vi "cam5_3dTest.vi"(7 "park plane z (px)":dbl=100.0, 8 "3d graph":refnum<k7>, 9 "transform cluster + actuator":T1, 10 "positions":T2, 11 "cells (image px locations)":dbl[][](array[numeric])=[[100.0, 300.0], [200.0, 400.0]]) -> (0 "current stage location (px)":dbl[](array[numeric]), 1 "current pipette locations (px)":dbl[][](array[numeric]), 2 "current cell locations (px)":dbl[][](array[numeric]), 3 "currentState out":T3(array[cluster]), 5 "current park plane z (px)":dbl=100.0)   [LabVIEW 2015]
uses:
  pipette cleaning/pressure box/cleaning_soft/controls/actuator_type.ctl
  pipette cleaning/pressure box/cleaning_soft/controls/actuator_cluster.ctl
  controls/transform_cluster_actuator.ctl
  transform_properties_actuators.ctl
panel:
  # "9/12/16\nUPDATES\n- real flag: show manipulator only if they are real"
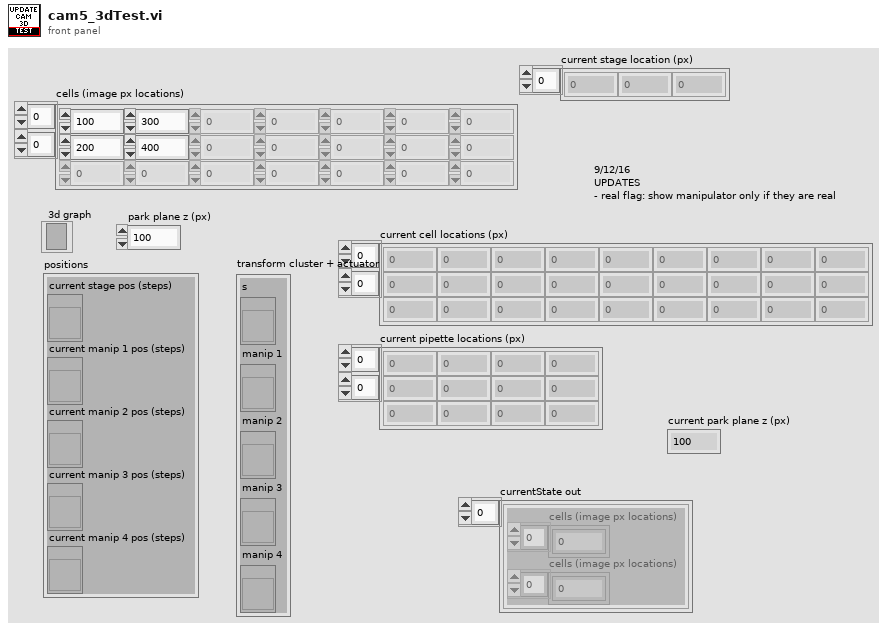
[diagram p1: front panel]
types:
  T1 = typedef "transform_cluster_actuator.ctl" = cluster{"s":refnum<vi>, "manip 1":refnum<vi>, "manip 2":refnum<vi>, "manip 3":refnum<vi>, "manip 4":refnum<vi>}
  T2 = cluster{"current stage pos (steps)":refnum<vi>, "current manip 1 pos (steps)":refnum<vi>, "current manip 2 pos (steps)":refnum<vi>, "current manip 3 pos (steps)":refnum<vi>, "current manip 4 pos (steps)":refnum<vi>}
  T3 = cluster{"cells (image px locations)":dbl[], "cells (image px locations)":dbl[]}[]
  T4 = typedef "transform_properties_actuators.ctl" = cluster{"theta (deg)":dbl, "X sc factor (px/step)":dbl, "Y sc factor (px/step)":dbl, "zero loc (x,y,z)":dbl[], "flip y?":bool, "flip x?":bool, "gamma (deg)":dbl, "flip z?":bool, "Z sc factor (px/step)":dbl, "actuator":T5, "safe space (steps)":i32[]}
  T5 = typedef "actuator_cluster.ctl" = cluster{"Actuator COM":refnum<visa-resource-name>, "Actuator type":T6}
  T6 = typedef "actuator_type.ctl" = enum16{"Scientifica", "Sutter", "Demo", "Off"}
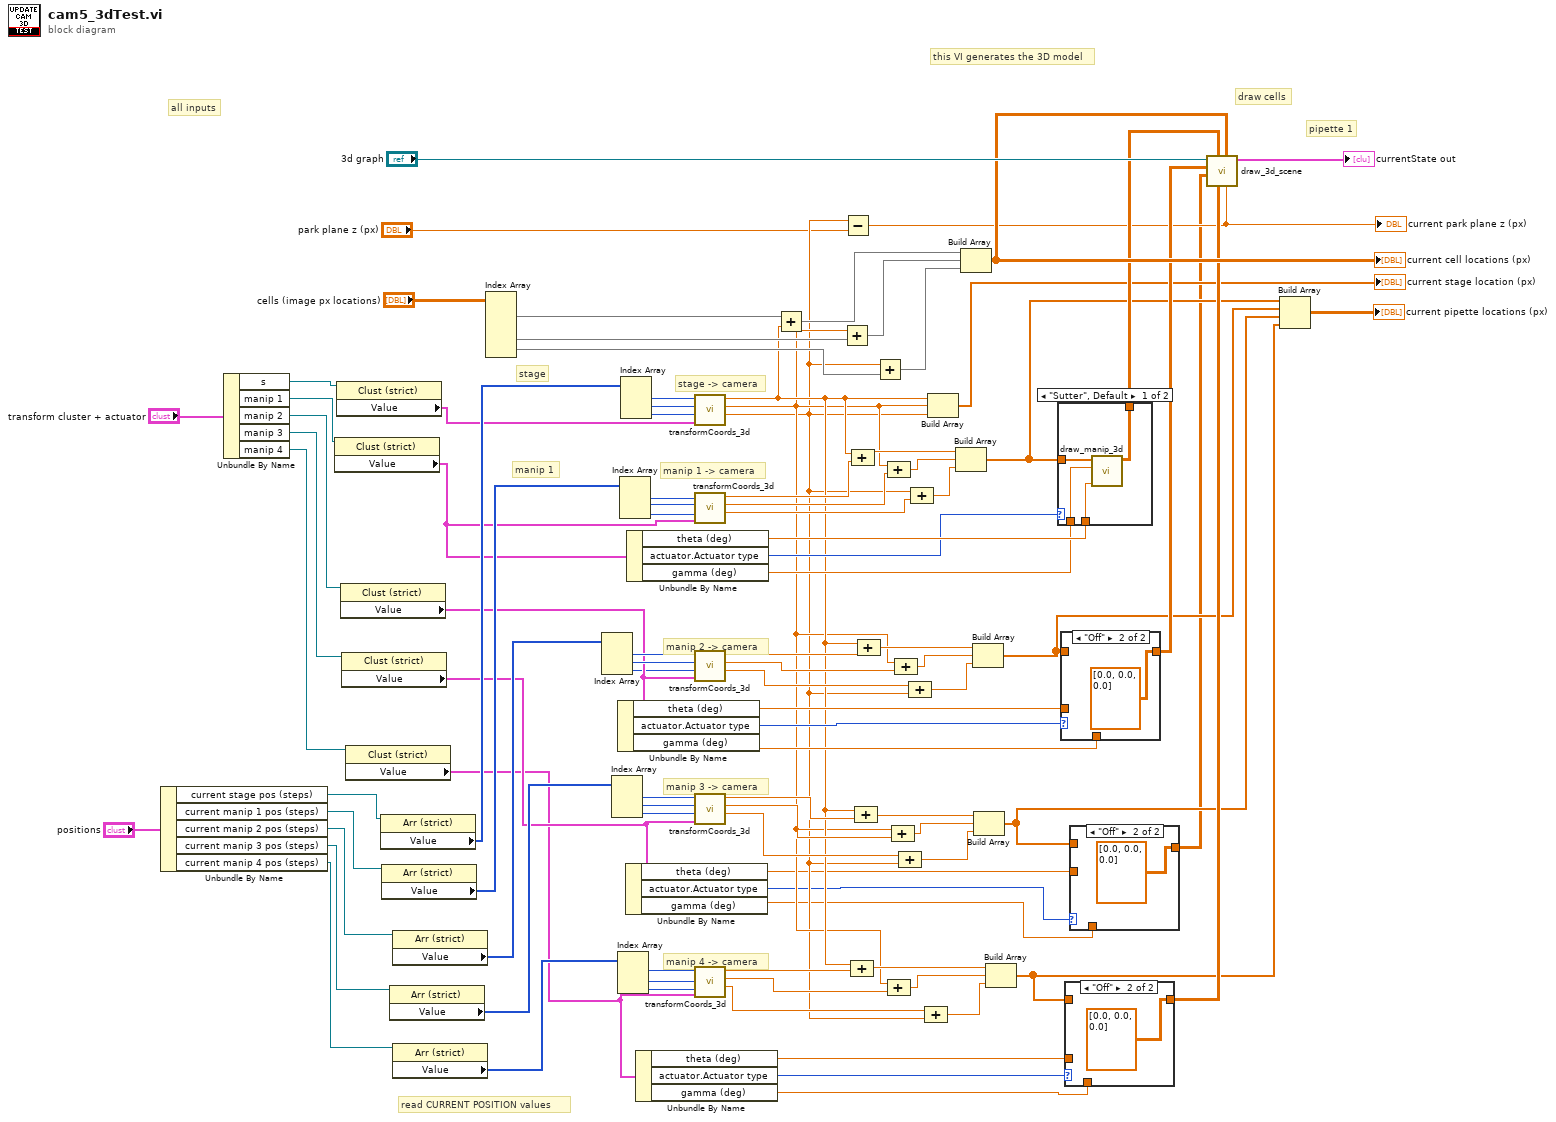
[diagram p0: block diagram]
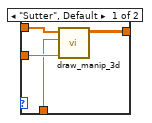
[diagram p2: hidden frame]
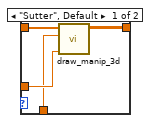
[diagram p3: hidden frame]
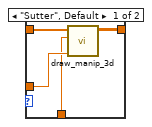
[diagram p4: hidden frame]
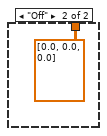
[diagram p5: hidden frame]
diagram:
  # "all inputs"
  # "this VI generates the 3D model"
  # "pipette 1"
  # "draw cells"
  # "manip 4 -> camera"
  # "manip 3 -> camera"
  # "manip 2 -> camera"
  # "manip 1 -> camera"
  # "manip 1"
  # "stage"
  # "read CURRENT POSITION values"
  # "stage -> camera"
  n1 = Unbundle By Name("positions") -> ("current stage pos (steps)"=w62:refnum<vi>, "current manip 1 pos (steps)"=w61:refnum<vi>, "current manip 2 pos (steps)"=w60:refnum<vi>, "current manip 3 pos (steps)"=w59:refnum<vi>, "current manip 4 pos (steps)"=w58:refnum<vi>)
  n2 = Unbundle By Name("transform cluster + actuator") -> ("s"=w16:refnum<vi>, "manip 1"=w55:refnum<vi>, "manip 2"=w54:refnum<vi>, "manip 3"=w53:refnum<vi>, "manip 4"=w52:refnum<vi>)
  n3 = property class="Clust (strict)"(reference=w55) -> ("Value"=w73:T4)  [unwired: 1 in, 2 out]
  n4 = property class="Clust (strict)"(reference=w16) -> ("Value"=w75:T4)  [unwired: 1 in, 2 out]
  n5 = property class="Clust (strict)"(reference=w54) -> ("Value"=w71:T4)  [unwired: 1 in, 2 out]
  n6 = property class="Clust (strict)"(reference=w53) -> ("Value"=w65:T4)  [unwired: 1 in, 2 out]
  n7 = property class="Clust (strict)"(reference=w52) -> ("Value"=w64:T4)  [unwired: 1 in, 2 out]
  n8 = property class="Arr (strict)"(reference=w62) -> ("Value"=w92:i32[])  [unwired: 1 in, 2 out]
  n9 = property class="Arr (strict)"(reference=w61) -> ("Value"=w91:i32[])  [unwired: 1 in, 2 out]
  n10 = property class="Arr (strict)"(reference=w59) -> ("Value"=w89:i32[])  [unwired: 1 in, 2 out]
  n11 = property class="Arr (strict)"(reference=w60) -> ("Value"=w90:i32[])  [unwired: 1 in, 2 out]
  n12 = property class="Arr (strict)"(reference=w58) -> ("Value"=w88:i32[])  [unwired: 1 in, 2 out]
  n13 = Index Array(array="cells (image px locations)") -> (element #1=w57:dbl[], element #2=w56:dbl[], element #3=w42:dbl[])  [unwired: 6 in]
  n14 = Index Array(array=w90) -> (element #1=w87:i32, element #2=w86:i32, element #3=w31:i32)  [unwired: 3 in]
  n15 = Index Array(array=w89) -> (element #1=w85:i32, element #2=w84:i32, element #3=w19:i32)  [unwired: 3 in]
  n16 = Unbundle By Name(w71) -> ("theta (deg)"=w66:dbl, "actuator.Actuator type"=w47:T6, "gamma (deg)"=w27:dbl)
  n17 = Index Array(array=w88) -> (element #1=w83:i32, element #2=w82:i32, element #3=w20:i32)  [unwired: 3 in]
  n18 = Index Array(array=w91) -> (element #1=w96:i32, element #2=w95:i32, element #3=w38:i32)  [unwired: 3 in]
  n19 = Index Array(array=w92) -> (element #1=w98:i32, element #2=w97:i32, element #3=w43:i32)  [unwired: 3 in]
  n20 = Unbundle By Name(w65) -> ("theta (deg)"=w1:dbl, "actuator.Actuator type"=w3:T6, "gamma (deg)"=w2:dbl)
  n21 = Unbundle By Name(w73) -> ("theta (deg)"=w72:dbl, "actuator.Actuator type"=w48:T6, "gamma (deg)"=w37:dbl)
  n22 = Unbundle By Name(w64) -> ("theta (deg)"=w63:dbl, "actuator.Actuator type"=w46:T6, "gamma (deg)"=w17:dbl)
  n23 = call "transformCoords_3d.vi"("transform properties"=w75, "z"=w43, "y"=w97, "x"=w98) -> ("z out"=w7:dbl, "y out"=w10:dbl, "x out"=w11:dbl)  [unwired: 5 in]
  n24 = call "transformCoords_3d.vi"("transform properties"=w73, "z"=w38, "y"=w95, "x"=w96) -> ("z out"=w39:dbl, "y out"=w93:dbl, "x out"=w94:dbl)  [unwired: 5 in]
  n25 = call "transformCoords_3d.vi"("transform properties"=w71, "z"=w31, "y"=w86, "x"=w87) -> ("z out"=w28:dbl, "y out"=w80:dbl, "x out"=w81:dbl)  [unwired: 5 in]
  n26 = call "transformCoords_3d.vi"("transform properties"=w65, "z"=w19, "y"=w84, "x"=w85) -> ("z out"=w24:dbl, "y out"=w78:dbl, "x out"=w79:dbl)  [unwired: 5 in]
  n27 = call "transformCoords_3d.vi"("transform properties"=w64, "z"=w20, "y"=w82, "x"=w83) -> ("z out"=w21:dbl, "y out"=w76:dbl, "x out"=w77:dbl)  [unwired: 5 in]
  n28 = Add(x=w57, y=w11) -> (x+y=w45:dbl[])
  n29 = Add(x=w10, y=w56) -> (x+y=w44:dbl[])
  n30 = Subtract(x=w7, y="park plane z (px)") -> (x-y=w8:dbl)
  "current park plane z (px)" <- w8
  n31 = Compound Arithmetic op=ADD(w11, w77) -> (w68:dbl)
  n32 = Compound Arithmetic op=ADD(w11, w94) -> (w74:dbl)
  n33 = Compound Arithmetic op=ADD(w11, w79) -> (w70:dbl)
  n34 = Compound Arithmetic op=ADD(w11, w81) -> (w67:dbl)
  n35 = Add(x=w7, y=w42) -> (x+y=w36:dbl[])
  n36 = Compound Arithmetic op=ADD(w10, w93) -> (w41:dbl)
  n37 = Compound Arithmetic op=ADD(w10, w76) -> (w23:dbl)
  n38 = Compound Arithmetic op=ADD(w10, w78) -> (w69:dbl)
  n39 = Compound Arithmetic op=ADD(w10, w80) -> (w30:dbl)
  n40 = Compound Arithmetic op=ADD(w24, w7) -> (w25:dbl)
  n41 = Compound Arithmetic op=ADD(w28, w7) -> (w29:dbl)
  n42 = Compound Arithmetic op=ADD(w7, w39) -> (w40:dbl)
  n43 = Compound Arithmetic op=ADD(w21, w7) -> (w22:dbl)
  n44 = Build Array(w11, w10, w7) -> (→"current stage location (px)":dbl[])
  n45 = Build Array(w74, w41, w40) -> (w15:dbl[])
  n46 = Build Array(w45, w44, w36) -> (w34:dbl[][])
  "current cell locations (px)" <- w34
  n47 = Build Array(w67, w30, w29) -> (w14:dbl[])
  n48 = Build Array(w70, w69, w25) -> (w5:dbl[])
  n49 = Build Array(w68, w23, w22) -> (w13:dbl[])
  n50 = case shown="\"Sutter\", Default" w48 {
    tunnel: w15 -> [w102 _]
    tunnel: w72 -> [w101 _]
    tunnel: w37 -> [w100 _]
    tunnel: [w99 dbl[][] [[0.0], [0.0], [0.0]] ("manip 3d location")] -> w32
    frame "Sutter", Default {
      n51 = call "draw_manip_3d.vi"("theta angle (deg)"=w101, "gamma angle (deg)"=w100, "manip tip coords"=w102) -> ("manip 3d location"=w99:dbl[][])  [unwired: 8 in]
    }
    frame "Off" {
    }
  }
  n52 = case shown="\"Off\"" w47 {
    tunnel: w14 -> [w107 _]
    tunnel: w66 -> [w106 _]
    tunnel: w27 -> [w105 _]
    tunnel: [w104 dbl[][] [[0.0], [0.0], [0.0]] ("manip 3d location")] -> w26
    frame "Sutter", Default {
      n53 = call "draw_manip_3d.vi"("theta angle (deg)"=w106, "gamma angle (deg)"=w105, "manip tip coords"=w107) -> ("manip 3d location"=w104:dbl[][])  [unwired: 8 in]
    }
    frame "Off" {
    }
  }
  n54 = case shown="\"Off\"" w46 {
    tunnel: w13 -> [w112 _]
    tunnel: w63 -> [w111 _]
    tunnel: [w110 dbl[][] [[0.0], [0.0], [0.0]] ("manip 3d location")] -> w18
    tunnel: w17 -> [w109 _]
    frame "Sutter", Default {
      n55 = call "draw_manip_3d.vi"("theta angle (deg)"=w111, "gamma angle (deg)"=w109, "manip tip coords"=w112) -> ("manip 3d location"=w110:dbl[][])  [unwired: 8 in]
    }
    frame "Off" {
    }
  }
  n56 = case shown="\"Off\"" w3 {
    tunnel: w5 -> [w117 _]
    tunnel: w1 -> [w116 _]
    tunnel: [w115 dbl[][] [[0.0], [0.0], [0.0]] ("manip 3d location")] -> w4
    tunnel: w2 -> [w114 _]
    frame "Sutter", Default {
      n57 = call "draw_manip_3d.vi"("theta angle (deg)"=w116, "gamma angle (deg)"=w114, "manip tip coords"=w117) -> ("manip 3d location"=w115:dbl[][])  [unwired: 8 in]
    }
    frame "Off" {
    }
  }
  n58 = call "draw_3d_scene.vi"("park plane z (px)"=w8, "cells"=w34, "manip 4"=w18, "manip 1"=w32, "manip 3"=w4, "manip 2"=w26, "3d graph"="3d graph") -> ("currentState out"=→"currentState out":T3)  [unwired: 3 in, 1 out]
  n59 = Build Array(w15, w14, w5, w13) -> (→"current pipette locations (px)":dbl[][])
